vi "Actor.vi"() -> (2 "Actor":refnum<class "Actor.lvclass">)   [LabVIEW 2025, in "_Template.lvlib" / "Templates.lvlib" / "TEMPLATE Actor.lvlib"]
uses:
  TEMPLATE Actor.lvlib
  jettl/jettl/Actor/Actor/Actor.lvclass
  TEMPLATE Actor/TEMPLATE Actor.lvclass
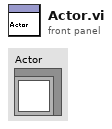
[diagram p1: front panel]
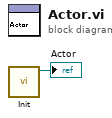
[diagram p0: block diagram]
diagram:
  n1 = call "Init.vi"() -> ("TEMPLATE Actor out"=→"Actor":refnum<class "TEMPLATE Actor.lvclass">)  [unwired: 11 in]
